vi "Online_SNR_Calculate.vi"(8 "error in (no error)":errorcluster, 11 "Online_SNR in":refnum<class "Online_SNR.lvclass">) -> (0 "error out":errorcluster, 3 "Online_SNR out":refnum<class "Online_SNR.lvclass">)   [LabVIEW 2021, in "Online_SNR.lvclass"]
uses:
  Online_SNR.lvclass
  Online_SNR.lvclass/Online_SNR.ctl
  Read Mean Square.vi
  Read Mean Square Error.vi
  Write SNR.vi
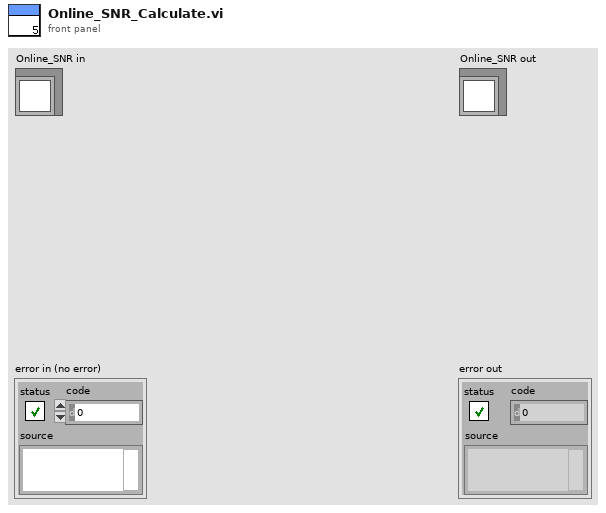
[diagram p1: front panel]
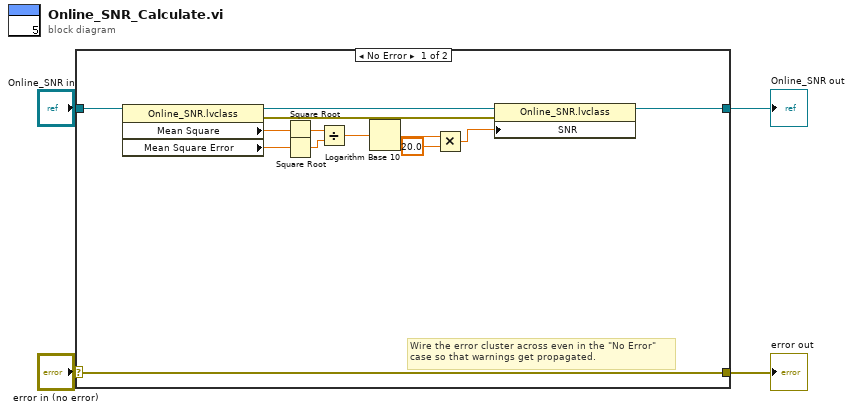
[diagram p0: block diagram]
diagram:
  n1 = case shown="No Error" "error in (no error)" {
    selector: "error in (no error)" -> [w17 w19]
    tunnel: [w17 w19] -> w3
    tunnel: [w13 w18] -> w1
    tunnel: "Online_SNR in" -> [w14 w18]
    frame No Error {
      # "Wire the error cluster across even in the \"No Error\"\ncase so that warnings get propagated."
      n2 = property class="Online_SNR.lvclass"(reference=w14) -> (reference out=w15:refnum<class "Online_SNR.lvclass">, error out=w16:errorcluster, "Mean Square"=w12:dbl, "Mean Square Error"=w11:dbl)  [unwired: 1 in]
      n3 = Square Root(x=w12) -> (sqrt(x)=w6:dbl)
      n4 = Square Root(x=w11) -> (sqrt(x)=w7:dbl)
      n5 = Divide(x=w6, y=w7) -> (x/y=w10:dbl)
      n6 = Logarithm Base 10(1:w10) -> (0:w9:dbl)
      n7 = Multiply(x=w9, y=20.0) -> (x*y=w5:dbl)
      n8 = property class="Online_SNR.lvclass"(reference=w15, error in=w16, "SNR"=w5) -> (reference out=w13:refnum<class "Online_SNR.lvclass">)  [unwired: 1 out]
    }
    frame Error {
    }
  }
  "error out" <- w3
  "Online_SNR out" <- w1
